vi "ISOSPI.vi"() -> ()   [LabVIEW 2020]
panel:
  in  "ISOSPI":string
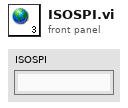
[diagram p1: front panel]
diagram:
